vi "TestCurveto.vi"(8 "error in (no error)":errorcluster) -> (0 "error out":errorcluster)   [LabVIEW 2019]
uses:
  PathCommands.CurveTo/PathCommands.CurveTo.lvclass
  PathCommands/Point.ctl
  <vilib>/addons/_JKI Toolkits/Caraya/classes/Assert/Assert Equal Value_Variant.vi
  <vilib>/addons/_JKI Toolkits/Caraya/classes/Assert/Assert False.vi
  <vilib>/addons/_JKI Toolkits/Caraya/classes/Assert/Assert True.vi
  <vilib>/addons/_JKI Toolkits/Caraya/classes/Test/Test.lvclass
  <vilib>/addons/_JKI Toolkits/Caraya/classes/Assert/Assert.lvclass
  PathCommands/PathCommands.lvclass
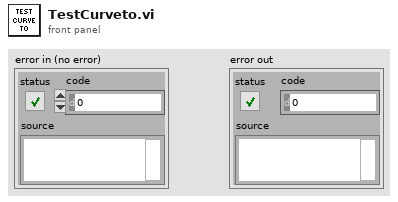
[diagram p1: front panel]
types:
  T1 = typedef "PathCommands.lvclass/Point.ctl" = cluster{"X":dbl, "Y":dbl}
  T2 = enum16{"None", "After", "Before", "Last", "First"}[]
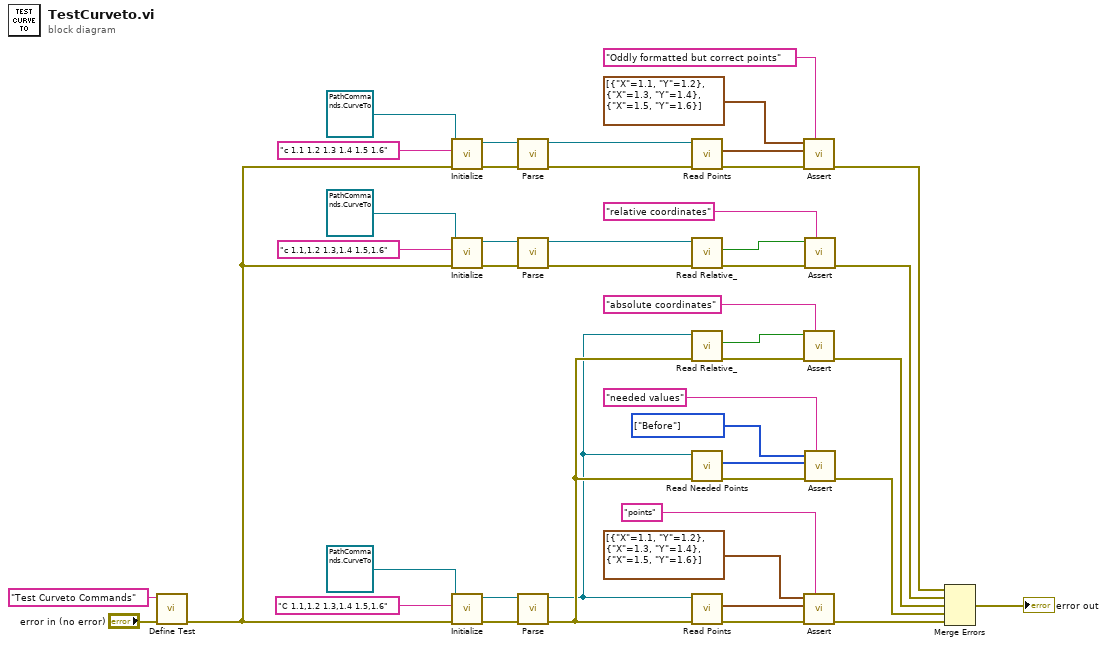
[diagram p0: block diagram]
diagram:
  w12 = T2 [enum."Before"] items=["None", "After", "Before", "Last", "First"] ("Needed Points 4")
  n1 = call <vilib>:"Define Test.vi"("error in (no error)"="error in (no error)", "Label (VI Title)"="Test Curveto Commands") -> ("error out"=w31:errorcluster)  [unwired: 8 in, 1 out]
  n2 = call-dynamic "Initialize.vi"("error in (no error)"=w31, "CommandText"="c 1.1 1.2 1.3 1.4 1.5 1.6", "PathCommands.CurveTo in"=refnum<class "PathCommands.CurveTo.lvclass"> refnum ("PathCommands.CurveTo.lvclass")) -> ("error out"=w32:errorcluster, "PathCommands.CurveTo out"=w5:refnum<class "PathCommands.CurveTo.lvclass">)  [unwired: 7 in]
  n3 = call-dynamic "Initialize.vi"("error in (no error)"=w31, "CommandText"="c 1.1,1.2 1.3,1.4 1.5,1.6", "PathCommands.CurveTo in"=refnum<class "PathCommands.CurveTo.lvclass"> refnum ("PathCommands.CurveTo.lvclass")) -> ("error out"=w38:errorcluster, "PathCommands.CurveTo out"=w17:refnum<class "PathCommands.CurveTo.lvclass">)  [unwired: 7 in]
  n4 = call-dynamic "Initialize.vi"("error in (no error)"=w31, "CommandText"="C 1.1,1.2 1.3,1.4 1.5,1.6", "PathCommands.CurveTo in"=refnum<class "PathCommands.CurveTo.lvclass"> refnum ("PathCommands.CurveTo.lvclass")) -> ("error out"=w44:errorcluster, "PathCommands.CurveTo out"=w24:refnum<class "PathCommands.CurveTo.lvclass">)  [unwired: 7 in]
  n5 = call-dynamic "Parse.vi"("error in (no error)"=w32, "PathCommands.CurveTo in"=w5) -> ("error out"=w34:errorcluster, "PathCommands.CurveTo out"=w9:refnum<class "PathCommands.CurveTo.lvclass">)  [unwired: 8 in]
  n6 = call-dynamic "Parse.vi"("error in (no error)"=w38, "PathCommands.CurveTo in"=w17) -> ("error out"=w40:errorcluster, "PathCommands.CurveTo out"=w20:refnum<class "PathCommands.CurveTo.lvclass">)  [unwired: 8 in]
  n7 = call-dynamic "Parse.vi"("error in (no error)"=w44, "PathCommands.CurveTo in"=w24) -> ("error out"=w35:errorcluster, "PathCommands.CurveTo out"=w10:refnum<class "PathCommands.CurveTo.lvclass">)  [unwired: 8 in]
  n8 = call-dynamic "Read Points.vi"("error in (no error)"=w34, "PathCommands in"=w9) -> ("error out"=w33:errorcluster, "Points"=w6:T1[])  [unwired: 7 in, 1 out]
  n9 = call-dynamic "Read Relative_.vi"("error in (no error)"=w40, "PathCommands in"=w20) -> ("error out"=w39:errorcluster, "Relative?"=w19:bool)  [unwired: 7 in, 1 out]
  n10 = call-dynamic "Read Relative_.vi"("error in (no error)"=w35, "PathCommands in"=w10) -> ("error out"=w37:errorcluster, "Relative?"=w14:bool)  [unwired: 7 in, 1 out]
  n11 = call-dynamic "Read Needed Points.vi"("error in (no error)"=w35, "PathCommands in"=w10) -> ("error out"=w36:errorcluster, "Needed Points"=w11:T2)  [unwired: 7 in, 1 out]
  n12 = call-dynamic "Read Points.vi"("error in (no error)"=w35, "PathCommands in"=w10) -> ("error out"=w43:errorcluster, "Points"=w23:T1[])  [unwired: 7 in, 1 out]
  n13 = call-poly <vilib>:"Assert.vi"("Label"="Oddly formatted but correct points", "error in (no error)"=w33, "Y"=w6, "X"=T1[] [{"X"=1.1, "Y"=1.2}, {"X"=1.3, "Y"=1.4}, {"X"=1.5, "Y"=1.6}] ("Points")) -> ("error out"=w27:errorcluster)  [unwired: 6 in, 1 out]
  n14 = call-poly <vilib>:"Assert.vi"("Label"="absolute coordinates", "error in (no error)"=w37, "False?"=w14) -> ("error out"=w29:errorcluster)  [unwired: 7 in, 1 out]
  n15 = call-poly <vilib>:"Assert.vi"("Label"="points", "error in (no error)"=w43, "Y"=w23, "X"=T1[] [{"X"=1.1, "Y"=1.2}, {"X"=1.3, "Y"=1.4}, {"X"=1.5, "Y"=1.6}] ("Points")) -> ("error out"=w41:errorcluster)  [unwired: 6 in, 1 out]
  n16 = call-poly <vilib>:"Assert.vi"("Label"="relative coordinates", "error in (no error)"=w39, "True?"=w19) -> ("error out"=w28:errorcluster)  [unwired: 7 in, 1 out]
  n17 = call-poly <vilib>:"Assert.vi"("Label"="needed values", "error in (no error)"=w36, "Y"=w11, "X"=w12) -> ("error out"=w30:errorcluster)  [unwired: 6 in, 1 out]
  n18 = Merge Errors(w27, w28, w29, w30, w41) -> (→"error out":errorcluster)
